vi "Page_Version_Initialize.vi"(6 "output cluster":T1, 8 "error in (no error)":errorcluster, 11 "AB_EXE in":refnum<class "AB_EXE.lvclass">) -> (0 "error out":errorcluster, 3 "AB_EXE out":refnum<class "AB_EXE.lvclass">)   [LabVIEW 2020, in "AB_EXE.lvclass"]
uses:
  <vilib>/AppBuilder/AB_Classes/EXE/AB_EXE.lvclass
  <resource>/Framework/Providers/Builds/AppBuilder/AB_UI_Page_Version_References.ctl
  <vilib>/AppBuilder/AB_Classes/Application/AB_Application.lvclass
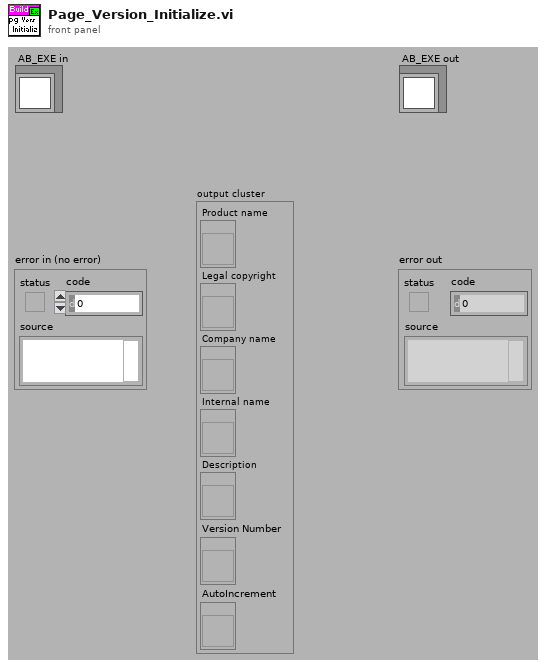
[diagram p1: front panel]
types:
  T1 = typedef "AB_UI_Page_Version_References.ctl" = cluster{"Product name":refnum<vi>, "Legal copyright":refnum<vi>, "Company name":refnum<vi>, "Internal name":refnum<vi>, "Description":refnum<vi>, "Version Number":refnum<vi>, "AutoIncrement":refnum<vi>}
  T2 = enum32{"invalid OS target", "Mac OS", "Windows 3.1", "Windows 95/NT", "Solaris 1", "Solaris 2", "HP-UX", "PowerMAX", "Linux", "Irix", "Rhapsody", "BeOS", "AIX", "OSF1", "VxWorks", "PharLap", "Carbon", "RTX", "Windows x64", "Linux x64", "Mac OS X x64"}
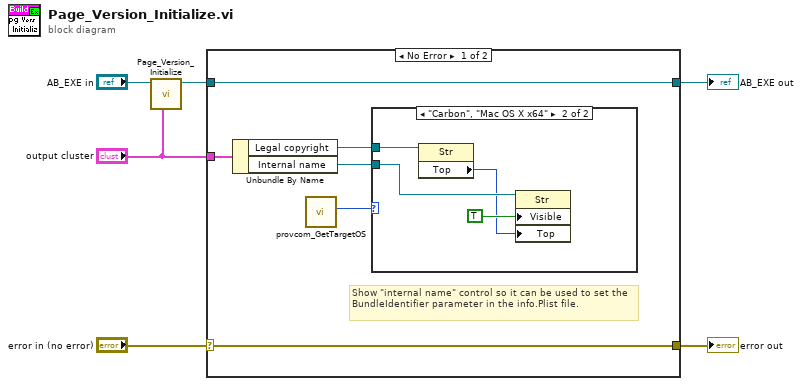
[diagram p0: block diagram]
diagram:
  n1 = call-parent "Page_Version_Initialize.vi"("output cluster"="output cluster", "AB_Targetfile in"="AB_EXE in") -> ("AB_Targetfile out"=w2:refnum<class "AB_EXE.lvclass">)  [unwired: 8 in, 1 out]
  n2 = case shown="No Error" "error in (no error)" {
    selector: "error in (no error)" -> [w11 w18]
    tunnel: [w11 w18] -> w4
    tunnel: [w12 w17] -> w6
    tunnel: w2 -> [w12 w17]
    tunnel: "output cluster" -> [w10 _]
    frame No Error {
      # "Show \"internal name\" control so it can be used to set the BundleIdentifier parameter in the info.Plist file."
      n3 = Unbundle By Name(w10) -> ("Legal copyright"=w8:refnum<vi>, "Internal name"=w7:refnum<vi>)
      n4 = call <resource>:"provcom_GetTargetOS.vi"() -> ("App.TargetOS"=w9:T2)  [unwired: 11 in]
      n5 = case shown="\"Carbon\", \"Mac OS X x64\"" w9 {
        tunnel: w8 -> [_ w14]
        tunnel: w7 -> [_ w16]
        frame Default {
        }
        frame "Carbon", "Mac OS X x64" {
          n6 = property class="Str"(reference=w14) -> ("Top"=w13:i32)  [unwired: 1 in, 2 out]
          n7 = property class="Str"(reference=w16, "Visible"=TRUE, "Top"=w13) -> ()  [unwired: 1 in, 2 out]
        }
      }
    }
    frame Error {
    }
  }
  "error out" <- w4
  "AB_EXE out" <- w6
